vi "Save File General Data Total Header.vi"(4 "Calibration Output Array":string[][](array[string]), 6 "File Name Output Array":string[][](array[string]), 7 "Save Data":string[][](array[string]), 8 "Error In":errorcluster, 9 "New File":bool, 10 "Data File Path In":path, 11 "First Call?: T/F":bool) -> (0 "Error Out":errorcluster, 1 "State (Adding Header (T), Else (F))":bool, 2 "Data After Initial":string[](array[string]), 3 "Initial Data Set":string[][](array[string]))   [LabVIEW 2020]
uses:
  <vilib>/Utility/file.llb/Write Delimited Spreadsheet (string).vi
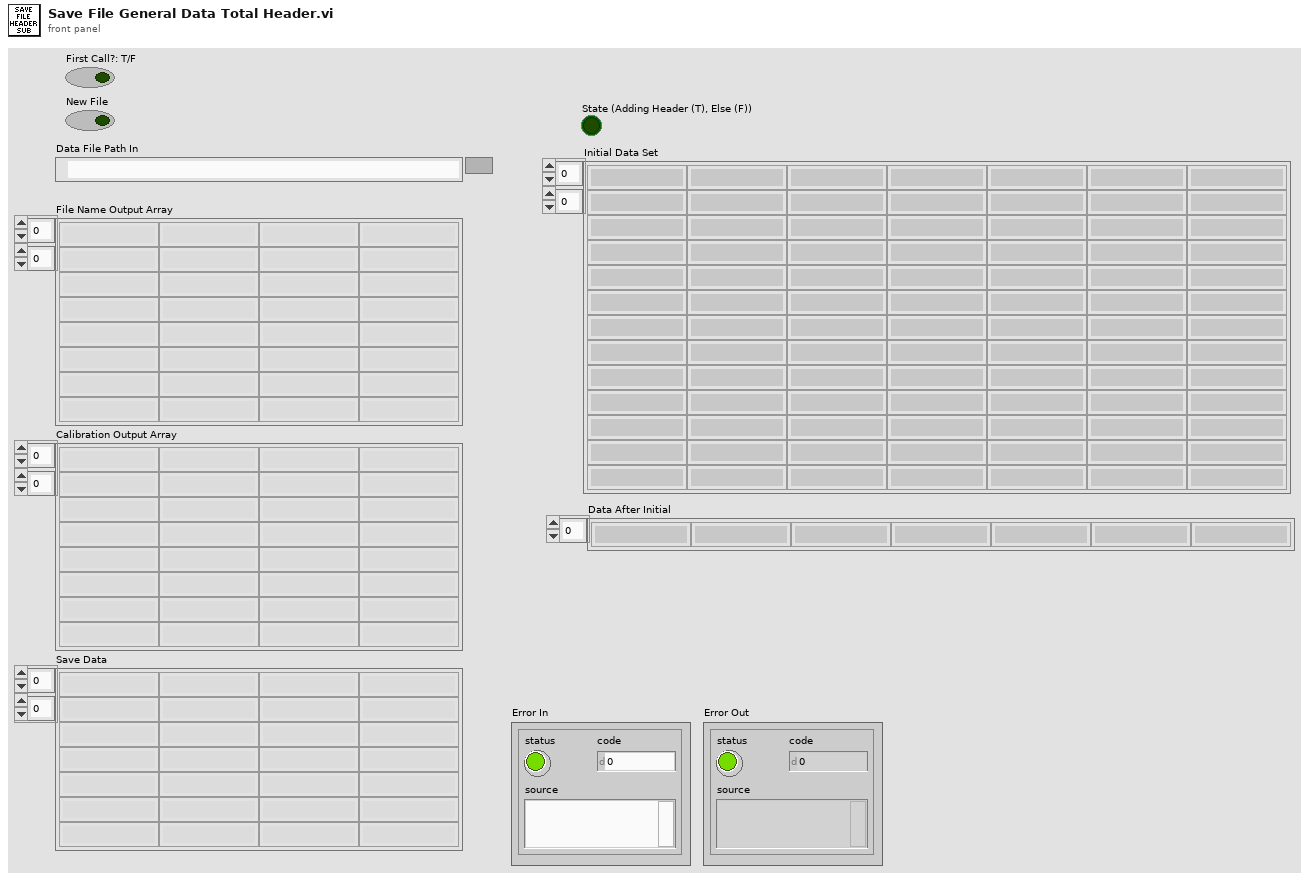
[diagram p1: front panel]
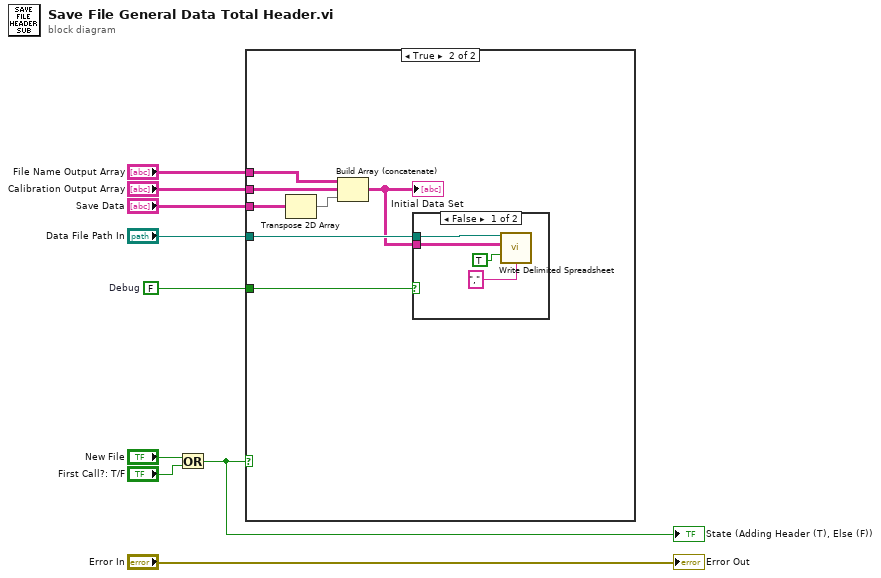
[diagram p0: block diagram]
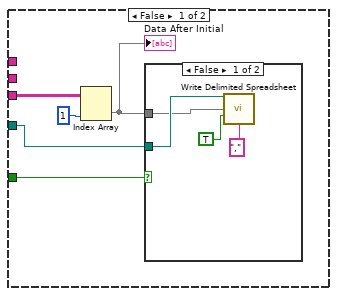
[diagram p2: hidden frame]
diagram:
  w1 = FALSE  # Debug
  n1 = Or(x="New File", y="First Call?: T/F") -> (x .or. y?=w3:bool)
  "State (Adding Header (T), Else (F))" <- w3
  n2 = case shown="True" w3 {
    tunnel: "File Name Output Array" -> [_ w25]
    tunnel: "Calibration Output Array" -> [_ w24]
    tunnel: "Save Data" -> [w13 w20]
    tunnel: "Data File Path In" -> [w14 w23]
    tunnel: w1 -> [w10 w21]
    frame False {
      n3 = Index Array(array=w13, index (col)=1 ("disabled index (col)")) -> (element=w11:string[])  [unwired: 1 in]
      "Data After Initial" <- w11
      n4 = case shown="False" w10 {
        tunnel: w14 -> [w18 _]
        tunnel: w11 -> [w15 _]
        frame False {
          n5 = call-poly <vilib>:"Write Delimited Spreadsheet.vi"("file path (dialog if empty)"=w18, "1D data"=w15, "append to file? (new file:F)"=TRUE, "delimiter (\\t)"="," ("delimiter (\\t)")) -> ()  [unwired: 10 in, 2 out]
        }
        frame True {
        }
      }
    }
    frame True {
      n6 = Transpose 2D Array(2D array=w20) -> (transposed array=w19:string[][])
      n7 = Build Array (concatenate)(w25, w24, w19) -> (w22:string[][])
      "Initial Data Set" <- w22
      n8 = case shown="False" w21 {
        tunnel: w23 -> [w29 _]
        tunnel: w22 -> [w26 _]
        frame False {
          n9 = call-poly <vilib>:"Write Delimited Spreadsheet.vi"("file path (dialog if empty)"=w29, "2D data"=w26, "append to file? (new file:F)"=TRUE, "delimiter (\\t)"="," ("delimiter (\\t)")) -> ()  [unwired: 10 in, 2 out]
        }
        frame True {
        }
      }
    }
  }
  "Error Out" <- "Error In"
